vi "reconnect.vi"(8 "error in (no error)":errorcluster, 11 "TCPServer in":refnum<class "TCPServer.lvclass">) -> (0 "error out":errorcluster, 3 "TCPServer out":refnum<class "TCPServer.lvclass">)   [LabVIEW 2016, in "TCPServer.lvclass"]
uses:
  TCPServer.lvclass
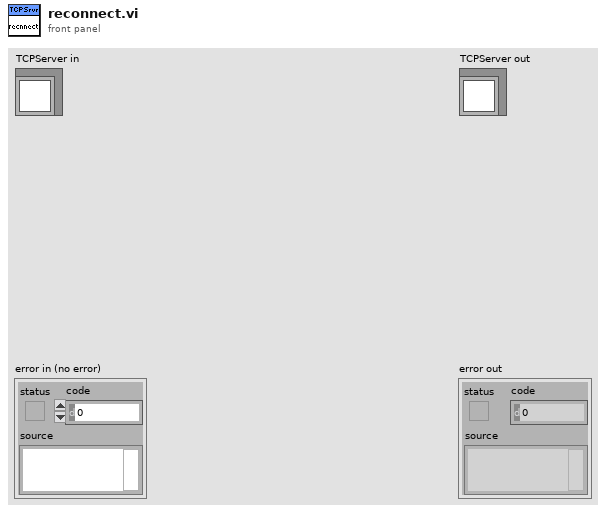
[diagram p1: front panel]
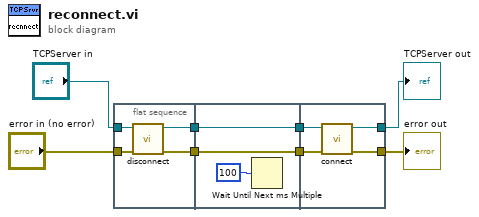
[diagram p0: block diagram]
diagram:
  n1 = flat-sequence {
    tunnel: [w11] -> w8
    tunnel: "error in (no error)" -> [w12]
    tunnel: "TCPServer in" -> [w10]
    tunnel: [w9] -> w3
    tunnel: w8 -> [w13]
    tunnel: [w14] -> w4
    tunnel: w3 -> [w14]
    tunnel: [w13] -> w2
    tunnel: [w18] -> w6
    tunnel: w4 -> [w17]
    tunnel: w2 -> [w19]
    tunnel: [w16] -> w1
    frame #0 {
      n2 = call-dynamic "disconnect.vi"("error in (no error)"=w12, "TCPServer in"=w10) -> ("error out"=w11:errorcluster, "TCPServer out"=w9:refnum<class "TCPServer.lvclass">)  [unwired: 8 in]
    }
    frame #1 {
      n3 = Wait Until Next ms Multiple(millisecond multiple=100) -> ()  [unwired: 1 out]
    }
    frame #2 {
      n4 = call-dynamic "connect.vi"("error in (no error)"=w19, "TCPServer in"=w17) -> ("error out"=w18:errorcluster, "TCPServer out"=w16:refnum<class "TCPServer.lvclass">)  [unwired: 8 in]
    }
  }
  "error out" <- w6
  "TCPServer out" <- w1
